vi "Hex Array to Str Hex Array.vi"(7 "Pre-Line Pad":string, 11 "Hex Array":u8[](array[numeric])) -> (3 "Hex Value String":string)   [LabVIEW 2026, in "LED Matrix.lvlib" / "LED Matrix.lvclass"]
uses:
  LED Matrix.lvclass
  LED Matrix.lvclass/LED Matrix.ctl
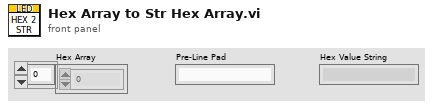
[diagram p1: front panel]
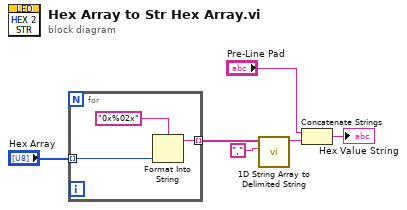
[diagram p0: block diagram]
diagram:
  n1 = for {
    tunnel: "Hex Array" -> [w9] mode=indexing
    tunnel: [w7] -> w4 mode=indexing
    n2 = Format Into String(format string="0x%02x", w9) -> (resulting string=w7:string)  [unwired: 2 in, 1 out]
  }
  n3 = call <vilib>:"1D String Array to Delimited String.vi"("delimiter"=",", "string array"=w4) -> ("delimited string"=w6:string)  [unwired: 9 in]
  n4 = Concatenate Strings("Pre-Line Pad", w6) -> (→"Hex Value String":string)
